vi "Valid Syntax List.vi"(0 "Message Popup in":refnum<class "Message Popup.lvclass">, 11 "error in (no error)":errorcluster) -> (4 "Message Popup out":refnum<class "Message Popup.lvclass">, 6 "Syntax List":T1[](array[typedef]), 15 "error out":errorcluster)   [LabVIEW 2016, in "Message Popup.lvclass"]
uses:
  Message Popup.lvclass
  common/Syntax Format.ctl
  common/Variable#.ctl
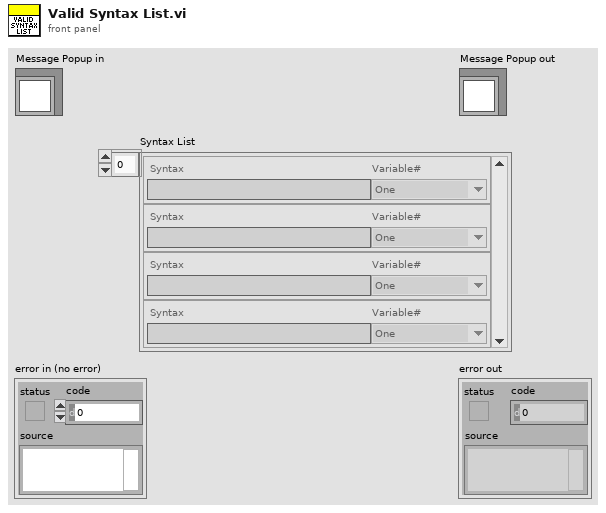
[diagram p1: front panel]
types:
  T1 = typedef "Syntax Format.ctl" = cluster{"Syntax":string, "Variable#":T2}
  T2 = typedef "Variable#.ctl" = enum16{"Zero", "One", "Two", "Three", "Four", "Five"}
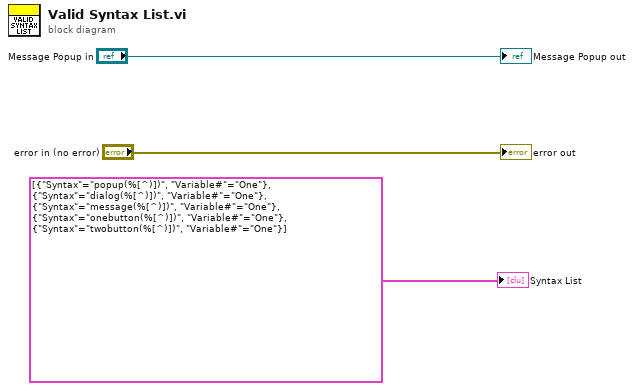
[diagram p0: block diagram]
diagram:
  "error out" <- "error in (no error)"
  "Message Popup out" <- "Message Popup in"
  "Syntax List" <- T1[] [{"Syntax"="popup(%[^)])", "Variable#"=enum."One"}, {"Syntax"="dialog(%[^)])", "Variable#"=enum."One"}, {"Syntax"="message(%[^)])", "Variable#"=enum."One"}, {"Syntax"="onebutton(%[^)])", "Variable#"=enum."One"}, {"Syntax"="twobutton(%[^)])", "Variable#"=enum."One"}] ("Syntax List")
